vi "FPGA Main.vi"() -> ()   [LabVIEW 2014]
uses:
  <vilib>/rvi/Emulation/niFpgaGetClockAttributes.vi
  <vilib>/rvi/Emulation/niFpgaSctlEmulationGetInTimedLoop.vi
  <vilib>/rvi/Emulation/niFpgaEmulationReportErrorSimple.vi
  <vilib>/rvi/eio/common/nirviEmuTemplateMethod_errors.vi
  <vilib>/rvi/Emulation/niFpgaCriticalErrorInLSC.vi
  <vilib>/rvi/interface/RandomDataEmulation/niFpgaRandomDataHandleErrors.vi
  <vilib>/eio/EIONode/EIONode.xnode
  <vilib>/rvi/DataTransferAndStorage/Container/XNode/niFpgaContainer.xnode
  <vilib>/rvi/interface/RandomDataEmulation/nirviRandomDataFpgaReadWriteTemplate.vi
panel:
  out "pH Exceed?":bool
  out "Temp Exceed?":bool
  in  "pH Threshold":sgl
  out "pHFIFOTimedOut?":bool
  out "TempFIFOTimedOut?":bool
  in  "Temp Threshold":sgl
  out "Simulator Timed Out?":bool
  in  "Siimulator Time out value":u32
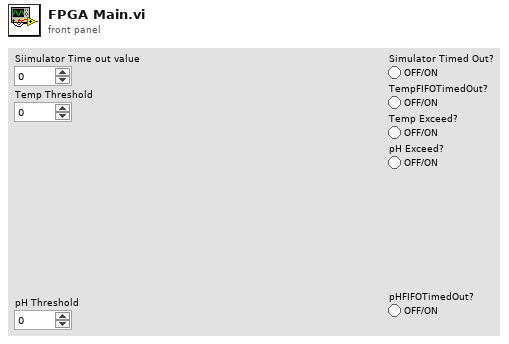
[diagram p1: front panel]
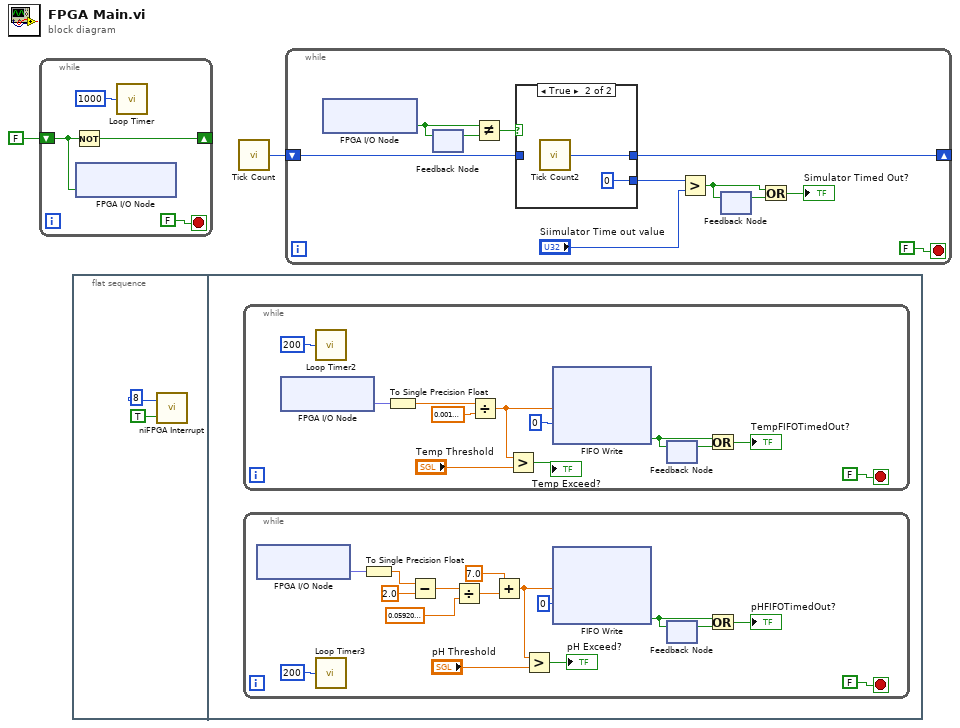
[diagram p0: block diagram]
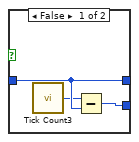
[diagram p2: hidden frame]
diagram:
  n1 = while {
    shift-right: [w3] -> _
    shift-left: FALSE -> [w4]
    stop <- FALSE stop-if-true
    n2 = Not(x=w4) -> (.not. x?=w3:bool)
    n3 = xnode "FPGA I/O Node"("Mod1/DO0"=w4) -> ()  [unwired: 1 in, 1 out]
    n4 = call "Loop Timer"("Count(mSec)"=u32 1000) -> ()  [unwired: 1 out]
  }
  n5 = flat-sequence {
    frame #0 {
      n6 = call <vilib>:"niFPGA Interrupt.vi"("Wait Until Cleared (F)"=TRUE, "IRQ Number (0)"=u8 8) -> ()  [unwired: 1 in]
    }
    frame #1 {
      n7 = while {
        stop <- FALSE stop-if-true
        n8 = xnode "FPGA I/O Node"() -> ("Mod4/AI0"=w36:fxp<+/-,16,5>)  [unwired: 1 in, 1 out]
        n9 = call "Loop Timer2"("Count(uSec)"=u32 200) -> ()  [unwired: 1 out]
        n10 = To Single Precision Float(number=w36) -> (single precision float=w35:sgl)
        n11 = Divide(x=w35, y=sgl 0.001) -> (x/y=w32:sgl)
        n12 = Greater?(x=w32, y="Temp Threshold") -> (0:→"Temp Exceed?":bool)
        n13 = xnode "FIFO Write"("Element"=w32, "Timeout"=0) -> ("Timed Out?"=w28:bool)  [unwired: 1 in, 1 out]
        n14 = feedback-in #1(w28) -> ()
        n15 = feedback #1() -> (w29:bool)  [unwired: 1 in]
        n16 = Or(x=w28, y=w29) -> (x .or. y?=→"TempFIFOTimedOut?":bool)
      }
      n17 = while {
        stop <- FALSE stop-if-true
        n18 = xnode "FPGA I/O Node"() -> ("Mod4/AI1"=w24:fxp<+/-,16,5>)  [unwired: 1 in, 1 out]
        n19 = call "Loop Timer3"("Count(uSec)"=u32 200) -> ()  [unwired: 1 out]
        n20 = To Single Precision Float(number=w24) -> (single precision float=w15:sgl)
        n21 = Subtract(x=w15, y=sgl 2.0) -> (x-y=w14:sgl)
        n22 = Divide(x=w14, y=sgl 0.0592) -> (x/y=w12:sgl)
        n23 = Add(x=sgl 7.0, y=w12) -> (x+y=w10:sgl)
        n24 = Greater?(x=w10, y="pH Threshold") -> (0:→"pH Exceed?":bool)
        n25 = xnode "FIFO Write"("Element"=w10, "Timeout"=0) -> ("Timed Out?"=w18:bool)  [unwired: 1 in, 1 out]
        n26 = feedback-in #2(w18) -> ()
        n27 = feedback #2() -> (w19:bool)  [unwired: 1 in]
        n28 = Or(x=w18, y=w19) -> (x .or. y?=→"pHFIFOTimedOut?":bool)
      }
    }
  }
  n29 = call "Tick Count"() -> ("Tick Count(mSec)"=w1:u32)
  n30 = while {
    shift-right: [w44] -> _
    shift-left: w1 -> [w43]
    stop <- FALSE stop-if-true
    n31 = xnode "FPGA I/O Node"() -> ("Mod2/DI0"=w46:bool)  [unwired: 1 in, 1 out]
    n32 = feedback-in #3(w46) -> ()
    n33 = feedback #3() -> (w47:bool)  [unwired: 1 in]
    n34 = Not Equal?(x=w46, y=w47) -> (x != y?=w45:bool)
    n35 = case shown="True" w45 {
      tunnel: [w50 w52] -> w44
      tunnel: w43 -> [w50 _]
      tunnel: [w48 u32 0] -> w42
      frame False {
        n36 = call "Tick Count3"() -> ("Tick Count(mSec)"=w49:u32)
        n37 = Subtract(x=w49, y=w50) -> (x-y=w48:u32)
      }
      frame True {
        n38 = call "Tick Count2"() -> ("Tick Count(mSec)"=w52:u32)
      }
    }
    n39 = Greater?(x=w42, y="Siimulator Time out value") -> (0:w40:bool)
    n40 = feedback-in #4(w40) -> ()
    n41 = feedback #4() -> (w39:bool)  [unwired: 1 in]
    n42 = Or(x=w40, y=w39) -> (x .or. y?=→"Simulator Timed Out?":bool)
  }
